vi "Test Connection Reset.vi"() -> ()   [LabVIEW 2016]
panel:
  out "General Settings:Resource Name":string
  out "read buffer":string
  in  "VISA resource name":refnum<visa-resource-name>
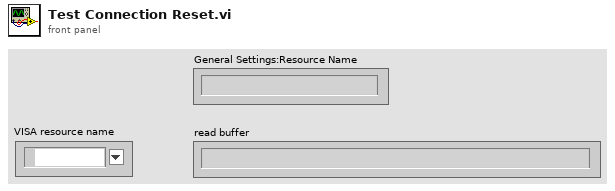
[diagram p1: front panel]
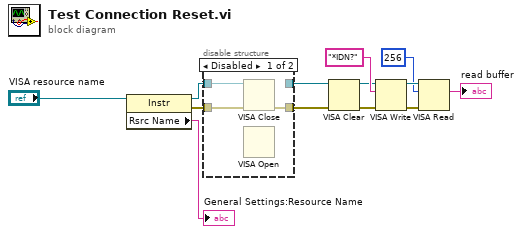
[diagram p0: block diagram]
diagram:
  n1 = property class="Instr"(reference="VISA resource name") -> (reference out=w7:refnum<visa-resource-name>, error out=w6:errorcluster, "Rsrc Name"=→"General Settings:Resource Name":string)  [unwired: 1 in]
  n2 = disable-structure shown="Disabled" {
    disable-tunnel: w7 -> [w16 w17]
    disable-tunnel: w6 -> [w15 w18]
    disable-tunnel: [w14 w18] -> w4
    disable-tunnel: [_ w17] -> w2
    frame Disabled {
      n3 = VISA Close(VISA resource name=w16, error in (no error)=w15) -> (error out=w14:errorcluster)
      n4 = VISA Open() -> ()  [unwired: 5 in, 2 out]
    }
    frame Enabled {
    }
  }
  n5 = VISA Clear(VISA resource name=w2, error in (no error)=w4) -> (VISA resource name out=w1:refnum<visa-resource-name>, error out=w3:errorcluster)
  n6 = VISA Write(VISA resource name=w1, write buffer="*IDN?", error in (no error)=w3) -> (VISA resource name out=w12:refnum<visa-resource-name>, error out=w11:errorcluster)  [unwired: 1 out]
  n7 = VISA Read(VISA resource name=w12, byte count=u32 256, error in (no error)=w11) -> (read buffer=→"read buffer":string)  [unwired: 3 out]
